vi "GetSimpleArray_SequentialRead.vi"(8 "error in":errorcluster, 9 "ArraySize":i32, 11 "node in":refnum<k20>) -> (0 "error out":errorcluster, 2 "TextArray":string[](array[string]), 3 "sibling node":refnum<k20>, 5 "node out":refnum<k20>)   [LabVIEW 2010, in "Pansino_XML_Read.lvlib"]
uses:
  <vilib>/xml/Close Reference(Node).vi
  Pansino_XML_Read.lvlib
  <vilib>/xml/NI_XML.lvlib
  C:/Program Files (x86)/National Instruments/LabVIEW 2010/resource/objmgr/DOMUserDefRef.rc
panel:
  out "Has Child Nodes":bool
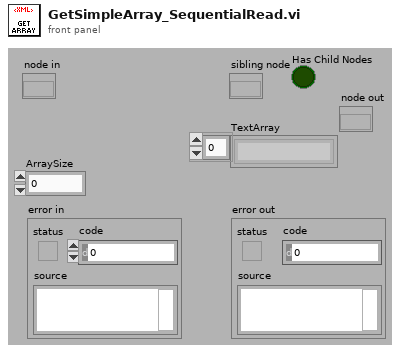
[diagram p1: front panel]
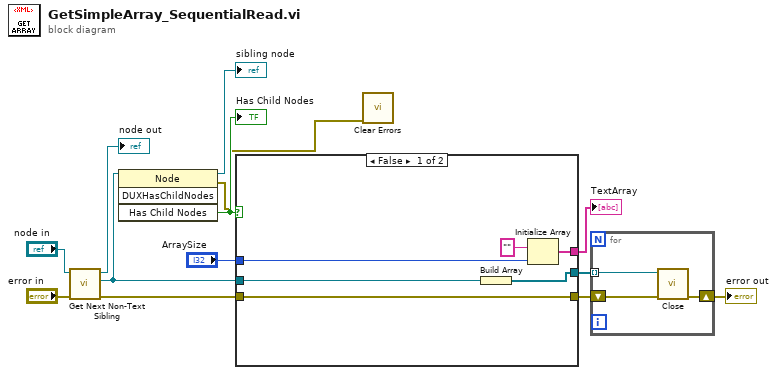
[diagram p0: block diagram]
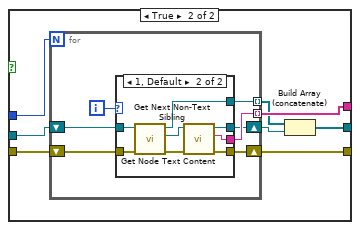
[diagram p2: hidden frame]
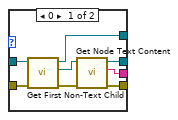
[diagram p3: hidden frame]
diagram:
  n1 = call <vilib>:"Get Next Non-Text Sibling.vi"("error in (no error)"="error in", "node in"="node in") -> ("error out"=w6:errorcluster, "sibling node"=w5:refnum<k20>, "node out"=→"node out":refnum<k20>)  [unwired: 7 out]
  n2 = invoke class="Node" method="DUXHasChildNodes"(reference=w5) -> (reference out=→"sibling node":refnum<k20>, error out=w1:errorcluster, "Has Child Nodes"=w10:bool)  [unwired: 3 in, 1 out]
  "Has Child Nodes" <- w10
  n3 = case shown="False" w10 {
    tunnel: [w14 w21] -> w9
    tunnel: [w19 w26] -> w8
    tunnel: "ArraySize" -> [w17 w25]
    tunnel: w5 -> [w18 w24]
    tunnel: w6 -> [w19 w23]
    tunnel: [w16 w22] -> w11
    frame False {
      n4 = Build Array(w18) -> (w14:refnum<k20>[])
      n5 = Initialize Array("" ("node text"), w17) -> (w16:string[])
    }
    frame True {
      n6 = for {
        N: w25 -> [_]
        tunnel: [w33] -> w22 mode=indexing
        shift-right: [w34] -> w26
        shift-left: w23 -> [w32]
        shift-right: [w30] -> w27
        shift-left: w24 -> [w31]
        tunnel: [w28] -> w20 mode=indexing
        i -> [w29]
        n7 = case shown="1, Default" w29 {
          tunnel: [w41 w49] -> w34
          tunnel: [w40 w48] -> w33
          tunnel: w32 -> [w37 w47]
          tunnel: w31 -> [w39 w46]
          tunnel: [w42 w45] -> w30
          tunnel: [w35 w43] -> w28
          frame 0 {
            n8 = call <vilib>:"Get First Non-Text Child.vi"("error in (no error)"=w37, "node in"=w39) -> ("error out"=w36:errorcluster, "child node"=w38:refnum<k20>, "node out"=w35:refnum<k20>)  [unwired: 6 in, 1 out]
            n9 = call <vilib>:"Get Node Text Content.vi"("error in (no error)"=w36, "node in"=w38) -> ("error out"=w41:errorcluster, "node text"=w40:string, "node out"=w42:refnum<k20>)  [unwired: 7 out]
          }
          frame 1, Default {
            n10 = call <vilib>:"Get Next Non-Text Sibling.vi"("error in (no error)"=w47, "node in"=w46) -> ("error out"=w44:errorcluster, "sibling node"=w50:refnum<k20>, "node out"=w43:refnum<k20>)  [unwired: 7 out]
            n11 = call <vilib>:"Get Node Text Content.vi"("error in (no error)"=w44, "node in"=w50) -> ("error out"=w49:errorcluster, "node text"=w48:string, "node out"=w45:refnum<k20>)  [unwired: 7 out]
          }
        }
      }
      n12 = Build Array (concatenate)(w20, w27) -> (w21:refnum<k20>[])
    }
  }
  "TextArray" <- w11
  n13 = call <vilib>:"Clear Errors.vi"("error in (no error)"=w1) -> ()  [unwired: 6 in, 1 out]
  n14 = for {
    tunnel: w9 -> [w52] mode=indexing
    shift-right: [w53] -> w13
    shift-left: w8 -> [w51]
    n15 = call-poly <vilib>:"Close.vi"("error in (no error)"=w51, "node"=w52) -> ("error out"=w53:errorcluster)  [unwired: 7 out]
  }
  "error out" <- w13
